vi "QuadEncActions.vi"(11 "Zero?":bool) -> (0 "RearRightQuadPos":i32, 1 "RearLeftQuadPos":i32, 2 "FrontRightQuadPos":i32, 3 "FrontLeftQuadPos":i32)   [LabVIEW 2018]
uses:
  <vilib>/Rock Robotics/WPI/ThirdParty/Phoenix-LabVIEW/Motor Controller/Get/CTRE_Phoenix_MotorController_GetQuadratureData.vi
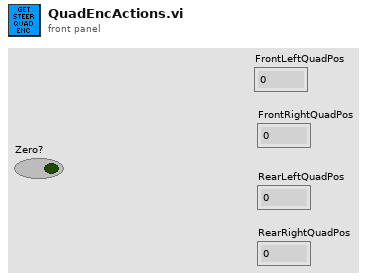
[diagram p1: front panel]
types:
  T1 = typedef "WPI_MotorControlDeviceRef.ctl" = cluster{"DeviceStatus":errorcluster, "Type":T2, "PWM":cluster{"PWM Channel":T3, "DeadBand":T4}, "CAN":cluster{"Device Number":u8, "SetOutput VI Ref":variant, "GetOutput VI Ref":variant, "Enable VI Ref":variant, "Disable VI Ref":variant, "Data":variant}, "Invert":bool, "DIO PWM":cluster{"PWM \"Enable\" Channel":T3, "DIOChannel":T5, "PWM Rate":dbl}}
  T2 = typedef "WPI_MotorControlType.ctl" = enum16{"PWM", "CAN", "DIO PWM"}
  T3 = typedef "FPGA_DIOPWMChannel.ctl" = enum8{"PWM 0", "PWM 1", "PWM 2", "PWM 3", "PWM 4", "PWM 5", "PWM 6", "PWM 7", "PWM 8", "PWM 9", "PWM MXP 0", "PWM MXP 1", "PWM MXP 2", "PWM MXP 3", "PWM MXP 4", "PWM MXP 5", "PWM MXP 6", "PWM MXP 7", "PWM MXP 8", "PWM MXP 9", "Invalid"}
  T4 = typedef "WPI_PWMDeadband.ctl" = cluster{"Name":string, "maxPositivePwm":i32, "minPositivePwm":i32, "centerPwm":i32, "maxNegativePwm":i32, "minNegativePwm":i32, "angularRange":u16}
  T5 = typedef "FPGA_DIOChannel.ctl" = enum8{"DIO 0", "DIO 1", "DIO 2", "DIO 3", "DIO 4", "DIO 5", "DIO 6", "DIO 7", "DIO 8", "DIO 9", "DIO MXP 0", "DIO MXP 1", "DIO MXP 2", "DIO MXP 3", "DIO MXP 4", "DIO MXP 5", "DIO MXP 6", "DIO MXP 7", "DIO MXP 8", "DIO MXP 9", "DIO MXP 10", "DIO MXP 11", "DIO MXP 12", "DIO MXP 13", "DIO MXP 14", "DIO MXP 15", "SPI Port CS1", "SPI Port CS2", "SPI Port CS3", "SPI Port MISO", "SPI Port MOSI", "Invalid"}
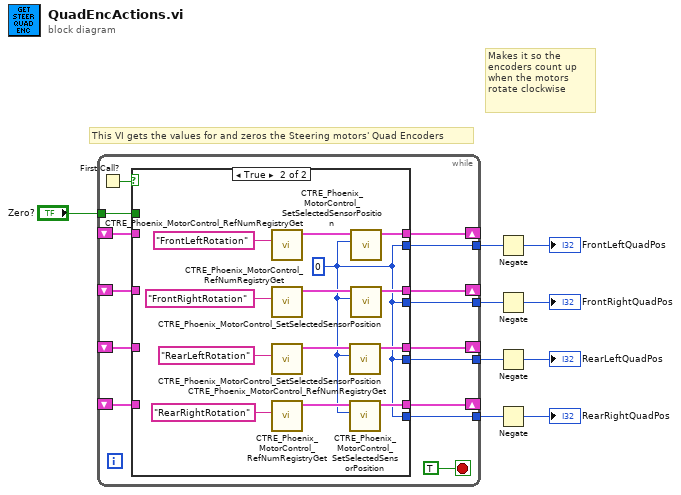
[diagram p0: block diagram]
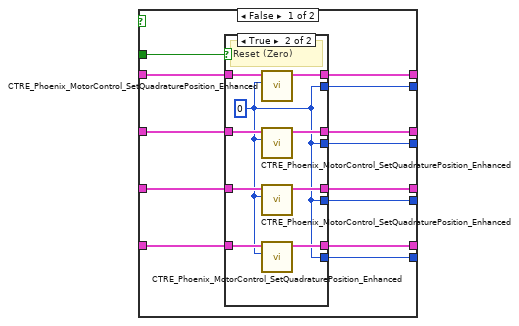
[diagram p2: hidden frame]
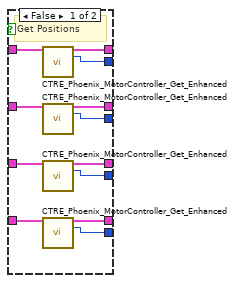
[diagram p3: hidden frame]
diagram:
  # "This VI gets the values for and zeros the Steering motors' Quad Encoders"
  # "Makes it so the encoders count up when the motors rotate clockwise"
  n1 = while {
    shift-right: [w23] -> _
    shift-left: _ -> [w22]
    shift-right: [w20] -> _
    shift-left: _ -> [w14]
    shift-right: [w18] -> _
    shift-left: _ -> [w13]
    shift-right: [w16] -> _
    shift-left: _ -> [w12]
    tunnel: [w24] -> w8
    tunnel: [w19] -> w2
    tunnel: [w17] -> w4
    tunnel: [w15] -> w6
    tunnel: "Zero?" -> [w10]
    stop <- TRUE stop-if-true
    n2 = First Call?() -> (First Call?: T/F=w21:bool)
    n3 = case shown="True" w21 {
      tunnel: w22 -> [w37 _]
      tunnel: [w36 w59] -> w24
      tunnel: [w35 w69] -> w23
      tunnel: [w33 w62] -> w20
      tunnel: [w28 w59] -> w19
      tunnel: [w32 w61] -> w18
      tunnel: [w27 w59] -> w17
      tunnel: [w29 w60] -> w16
      tunnel: [w26 w59] -> w15
      tunnel: w14 -> [w34 _]
      tunnel: w13 -> [w31 _]
      tunnel: w12 -> [w30 _]
      tunnel: w10 -> [w25 _]
      frame False {
        n4 = case shown="True" w25 {
          tunnel: w37 -> [w49 w58]
          tunnel: [w48 w50] -> w36
          tunnel: [w47 w57] -> w35
          tunnel: w34 -> [w46 w56]
          tunnel: [w45 w55] -> w33
          tunnel: [w44 w53] -> w32
          tunnel: w31 -> [w43 w54]
          tunnel: w30 -> [w42 w51]
          tunnel: [w41 w52] -> w29
          tunnel: [w40 w50] -> w28
          tunnel: [w39 w50] -> w27
          tunnel: [w38 w50] -> w26
          frame False {
            # "Get Positions"
            n5 = call-poly <vilib>:"CTRE_Phoenix_MotorController_Get_Enhanced.vi"("PhoenixMotorControlDevRef"=w49) -> ("PhoenixMotorControlDevRef"=w47:T1, "Quadrature Position"=w48:i32)  [unwired: 11 in, 2 out]
            n6 = call-poly <vilib>:"CTRE_Phoenix_MotorController_Get_Enhanced.vi"("PhoenixMotorControlDevRef"=w46) -> ("PhoenixMotorControlDevRef"=w45:T1, "Quadrature Position"=w40:i32)  [unwired: 11 in, 2 out]
            n7 = call-poly <vilib>:"CTRE_Phoenix_MotorController_Get_Enhanced.vi"("PhoenixMotorControlDevRef"=w43) -> ("PhoenixMotorControlDevRef"=w44:T1, "Quadrature Position"=w39:i32)  [unwired: 11 in, 2 out]
            n8 = call-poly <vilib>:"CTRE_Phoenix_MotorController_Get_Enhanced.vi"("PhoenixMotorControlDevRef"=w42) -> ("PhoenixMotorControlDevRef"=w41:T1, "Quadrature Position"=w38:i32)  [unwired: 11 in, 2 out]
          }
          frame True {
            w50 = 0 ("New Position")
            # "Reset (Zero)"
            n9 = call <vilib>:"CTRE_Phoenix_MotorControl_SetQuadraturePosition_Enhanced.vi"("New Position"=w50, "PhoenixMotorControlDevRef"=w58) -> ("PhoenixMotorControlDevRef"=w57:T1)  [unwired: 8 in, 1 out]
            n10 = call <vilib>:"CTRE_Phoenix_MotorControl_SetQuadraturePosition_Enhanced.vi"("New Position"=w50, "PhoenixMotorControlDevRef"=w56) -> ("PhoenixMotorControlDevRef"=w55:T1)  [unwired: 8 in, 1 out]
            n11 = call <vilib>:"CTRE_Phoenix_MotorControl_SetQuadraturePosition_Enhanced.vi"("New Position"=w50, "PhoenixMotorControlDevRef"=w54) -> ("PhoenixMotorControlDevRef"=w53:T1)  [unwired: 8 in, 1 out]
            n12 = call <vilib>:"CTRE_Phoenix_MotorControl_SetQuadraturePosition_Enhanced.vi"("New Position"=w50, "PhoenixMotorControlDevRef"=w51) -> ("PhoenixMotorControlDevRef"=w52:T1)  [unwired: 8 in, 1 out]
          }
        }
      }
      frame True {
        w59 = 0 ("New Sensor Position")
        n13 = call <vilib>:"CTRE_Phoenix_MotorControl_RefNumRegistryGet.vi"("refnum name"="FrontLeftRotation") -> ("PhoenixMotorControlDevRef"=w70:T1)  [unwired: 9 in, 1 out]
        n14 = call <vilib>:"CTRE_Phoenix_MotorControl_RefNumRegistryGet.vi"("refnum name"="FrontRightRotation") -> ("PhoenixMotorControlDevRef"=w68:T1)  [unwired: 9 in, 1 out]
        n15 = call <vilib>:"CTRE_Phoenix_MotorControl_RefNumRegistryGet.vi"("refnum name"="RearLeftRotation") -> ("PhoenixMotorControlDevRef"=w65:T1)  [unwired: 9 in, 1 out]
        n16 = call <vilib>:"CTRE_Phoenix_MotorControl_RefNumRegistryGet.vi"("refnum name"="RearRightRotation") -> ("PhoenixMotorControlDevRef"=w64:T1)  [unwired: 9 in, 1 out]
        n17 = call <vilib>:"CTRE_Phoenix_MotorControl_SetSelectedSensorPosition.vi"("New Sensor Position"=w59, "PhoenixMotorControlDevRef"=w65) -> ("PhoenixMotorControlDevRef"=w61:T1)  [unwired: 8 in, 1 out]
        n18 = call <vilib>:"CTRE_Phoenix_MotorControl_SetSelectedSensorPosition.vi"("New Sensor Position"=w59, "PhoenixMotorControlDevRef"=w64) -> ("PhoenixMotorControlDevRef"=w60:T1)  [unwired: 8 in, 1 out]
        n19 = call <vilib>:"CTRE_Phoenix_MotorControl_SetSelectedSensorPosition.vi"("New Sensor Position"=w59, "PhoenixMotorControlDevRef"=w70) -> ("PhoenixMotorControlDevRef"=w69:T1)  [unwired: 8 in, 1 out]
        n20 = call <vilib>:"CTRE_Phoenix_MotorControl_SetSelectedSensorPosition.vi"("New Sensor Position"=w59, "PhoenixMotorControlDevRef"=w68) -> ("PhoenixMotorControlDevRef"=w62:T1)  [unwired: 8 in, 1 out]
      }
    }
  }
  n21 = Negate(x=w8) -> (-x=→"FrontLeftQuadPos":i32)
  n22 = Negate(x=w2) -> (-x=→"FrontRightQuadPos":i32)
  n23 = Negate(x=w4) -> (-x=→"RearLeftQuadPos":i32)
  n24 = Negate(x=w6) -> (-x=→"RearRightQuadPos":i32)
